vi "to_variant.vi"(8 "error in (no error)":errorcluster, 11 "LVData in":refnum<class "LVData.lvclass">) -> (0 "error out":errorcluster, 3 "Data out":variant)   [LabVIEW 2020, in "lvdata.lvlib" / "LVData.lvclass"]
uses:
  LVData.lvclass
  LVData.lvclass/LVData.ctl
  Bytes/Bytes.lvclass/Bytes.ctl
  DataString/DataString.lvclass
  C:/projects/OpenG-Variant-Data-Library/source/library/Bytes/Bytes.lvclass
  Type Descriptor/TypeDescriptor.lvclass
  Bytes/Bytes.lvclass
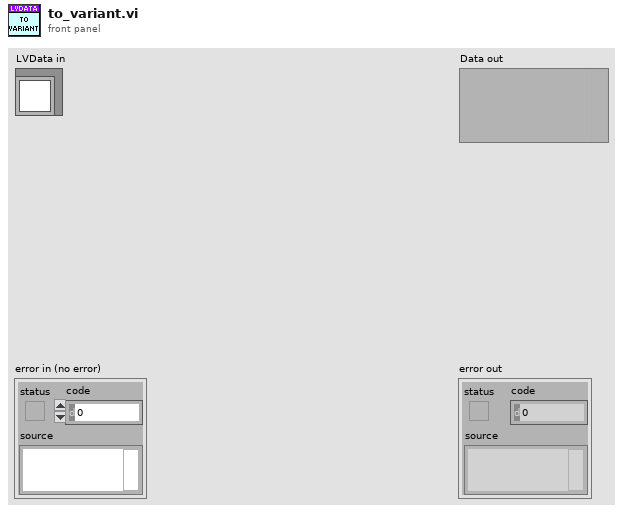
[diagram p1: front panel]
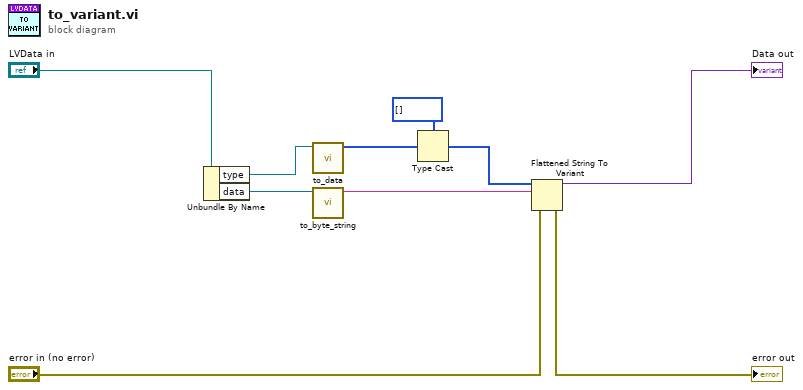
[diagram p0: block diagram]
diagram:
  n1 = Unbundle By Name("LVData in") -> ("type"=w9:refnum<class "TypeDescriptor.lvclass">, "data"=w10:refnum<class "DataString.lvclass">)
  n2 = call "to_data.vi"("Bytes in"=w9) -> ("byte array"=w7:u8[])  [unwired: 10 in]
  n3 = call "to_byte_string.vi"("Bytes in"=w10) -> ("byte string"=w8:string)  [unwired: 10 in]
  n4 = Type Cast(type=i16[] [] ("type string"), x=w7) -> (*(type *) &x=w5:i16[])
  n5 = Flattened String To Variant(4:"error in (no error)", 6:w8, 7:w5) -> (0:→"error out":errorcluster, 3:→"Data out":variant)
